vi "select_max_spectrum.vi"(9 "window freq":dbl, 10 "index":i32, 11 "psd data":cluster{"f0":dbl, "df":dbl, "magnitude":dbl[]}) -> (1 "noise":cluster{"f0":dbl, "df":dbl, "magnitude":dbl[]}(graph), 2 "signal":cluster{"f0":dbl, "df":dbl, "magnitude":dbl[]}(graph), 3 "whole":cluster{"f0":dbl, "df":dbl, "magnitude":dbl[]}(graph))   [LabVIEW 2017]
panel:
  out "PSD":cluster{"f0":dbl, "df":dbl, "magnitude":dbl[]}[](graph)
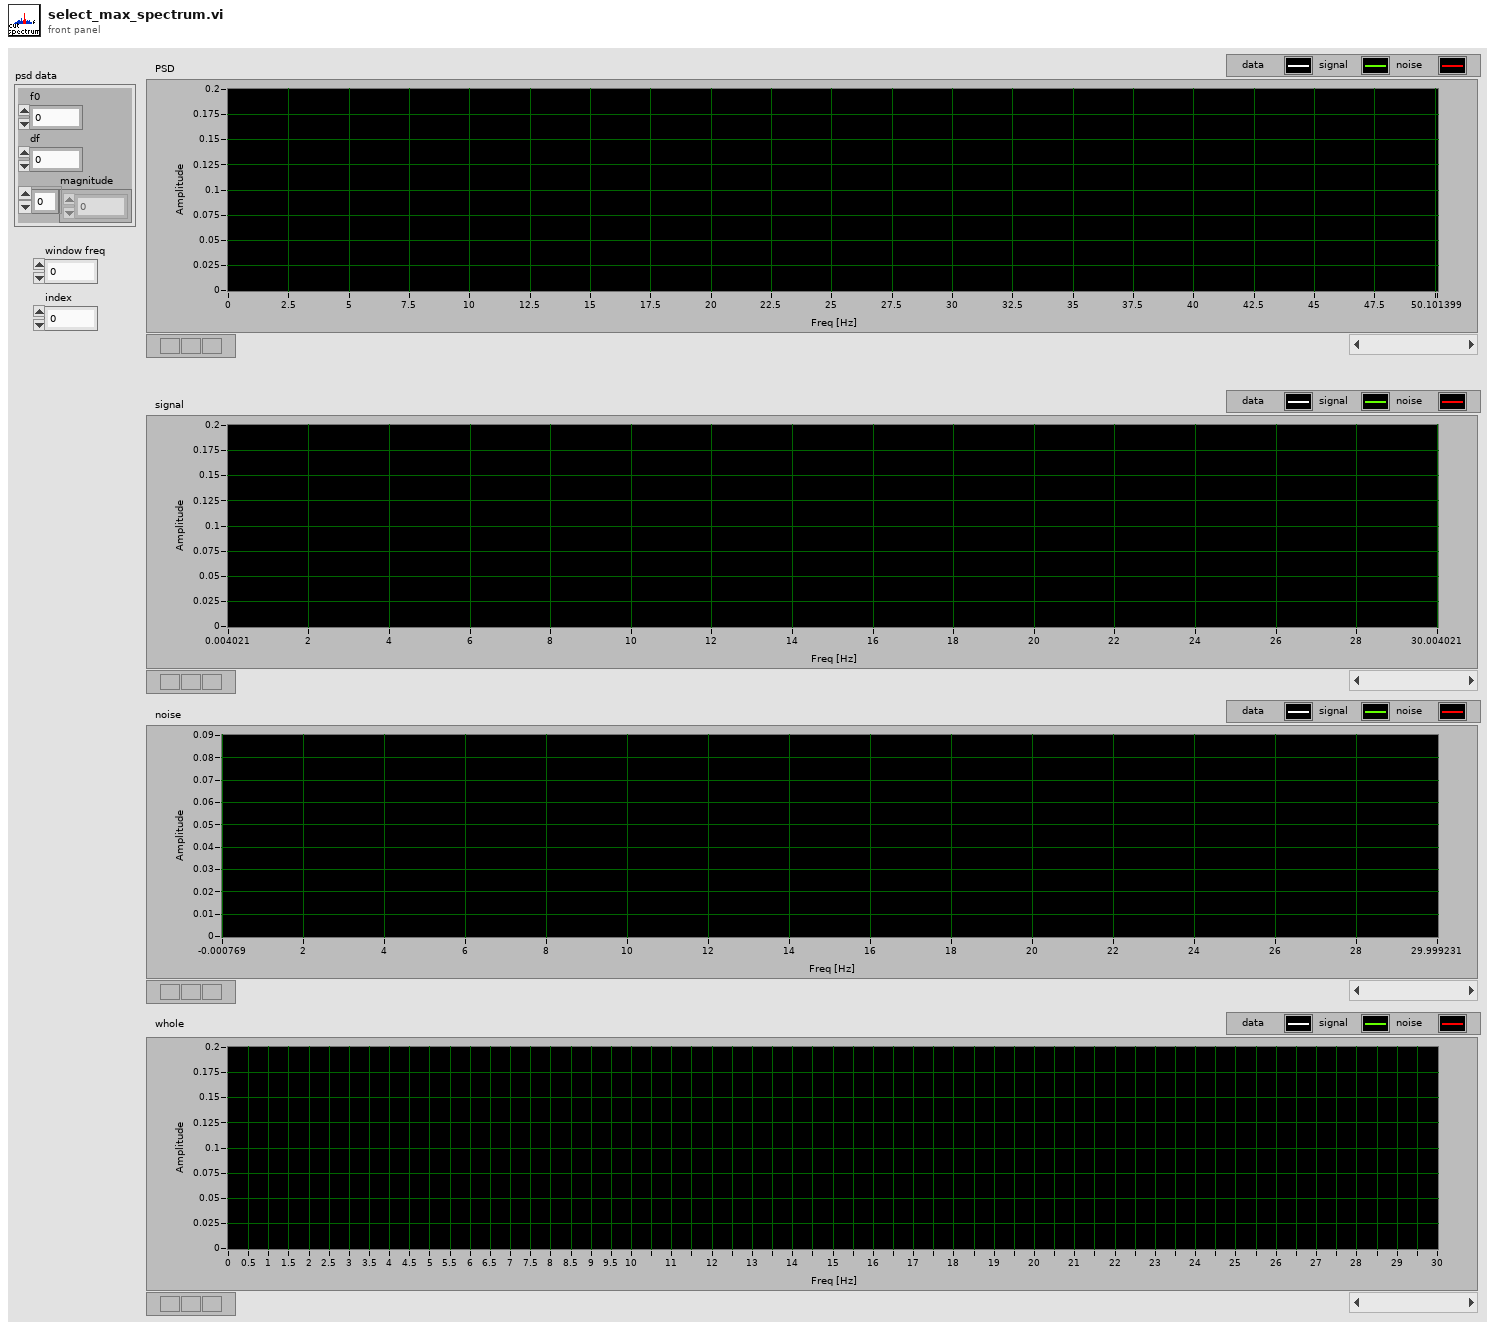
[diagram p1: front panel]
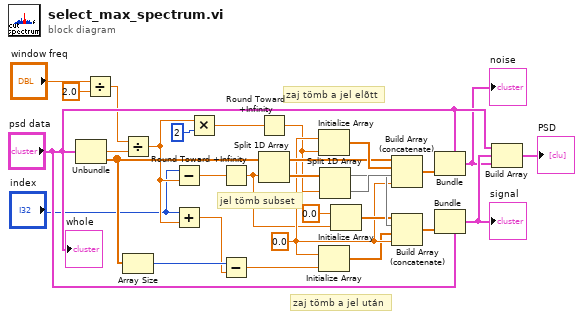
[diagram p0: block diagram]
diagram:
  w17 = 0.0 ("element")
  # "zaj tömb a jel után"
  # "zaj tömb a jel elõtt"
  # "jel tömb subset"
  n1 = Unbundle("psd data") -> ("df"=w7:dbl, "magnitude"=w15:dbl[])  [unwired: 1 out]
  n2 = Divide(x="window freq", y=2.0) -> (x/y=w8:dbl)
  n3 = Divide(x=w8, y=w7) -> (x/y=w6:dbl)
  n4 = Array Size(array=w15) -> (size(s)=w20:i32)
  n5 = Subtract(x="index", y=w6) -> (x-y=w5:dbl)
  n6 = Add(x="index", y=w6) -> (x+y=w19:dbl)
  n7 = Multiply(x=w6, y=2) -> (x*y=w3:dbl)
  n8 = Round Toward +Infinity(x=w5) -> (ceil(x): smallest int >= x=w4:dbl)
  n9 = Subtract(x=w20, y=w19) -> (x-y=w18:dbl)
  n10 = Round Toward +Infinity(x=w3) -> (ceil(x): smallest int >= x=w2:dbl)
  n11 = Split 1D Array(array=w15, index=w4) -> (first subarray=w26:dbl[], second subarray=w29:dbl[])
  n12 = Initialize Array "Initialize Array"(w17, w2) -> (w27:dbl[])
  n13 = Initialize Array(w17, w18) -> (w16:dbl[])
  n14 = Split 1D Array(array=w29, index=w2) -> (first subarray=w24:dbl[], second subarray=w25:dbl[])
  n15 = Initialize Array(0.0 ("element"), w4) -> (w22:dbl[])
  n16 = Build Array (concatenate)(w26, w27, w25, w17) -> (w28:dbl[])
  n17 = Build Array (concatenate)(w22, w24, w16, w17) -> (w21:dbl[])
  n18 = Bundle(cluster="psd data", "magnitude"=w28) -> (w10:cluster{"f0":dbl, "df":dbl, "magnitude":dbl[]})  [unwired: 2 in]
  "noise" <- w10
  n19 = Bundle(cluster="psd data", "magnitude"=w21) -> (w12:cluster{"f0":dbl, "df":dbl, "magnitude":dbl[]})  [unwired: 2 in]
  "signal" <- w12
  n20 = Build Array("psd data", w12, w10) -> (→"PSD":cluster{"f0":dbl, "df":dbl, "magnitude":dbl[]}[])
  "whole" <- "psd data"
